vi "delete channel from configuration.vi"(8 "error in":errorcluster, 10 "channel":refnum<class "TBM channel.lvclass">, 11 "Scaling configuration in":refnum<class "Scaling configuration.lvclass">) -> (0 "error out":errorcluster, 3 "Scaling configuration out":refnum<class "Scaling configuration.lvclass">)   [LabVIEW 2013, in "Scaling configuration.lvclass"]
uses:
  Scaling configuration.lvclass
  <vilib>/NI/Tag Bus Module Framework/channel/TBM channel.lvclass
  <vilib>/NI/Tag Bus/tag/tag descriptor.lvclass
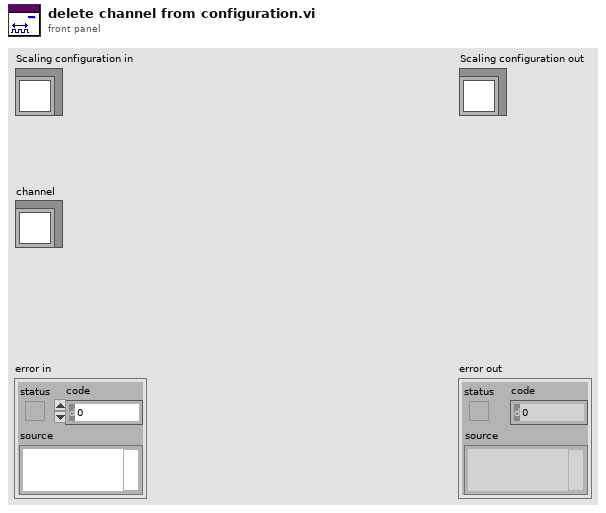
[diagram p1: front panel]
types:
  T1 = typedef "Scaling configuration.lvclass/scale data types.ctl" = enum16{"Double", "Single", "I64", "I32", "I16", "I8", "U64", "U32", "U16", "U8"}
  T2 = cluster{"input channel":refnum<class "TBM channel.lvclass">, "output channel":refnum<class "TBM channel.lvclass">, "input data type":T1, "output data type":T1}[][]
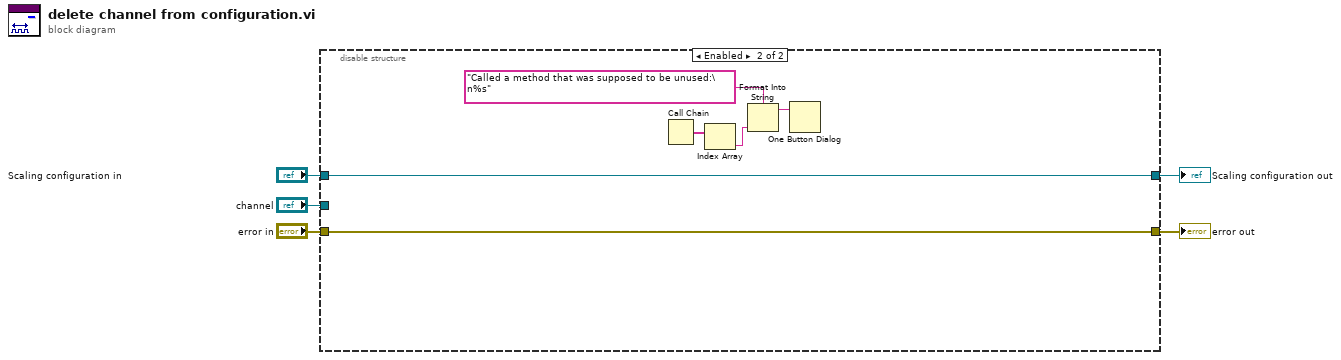
[diagram p0: block diagram]
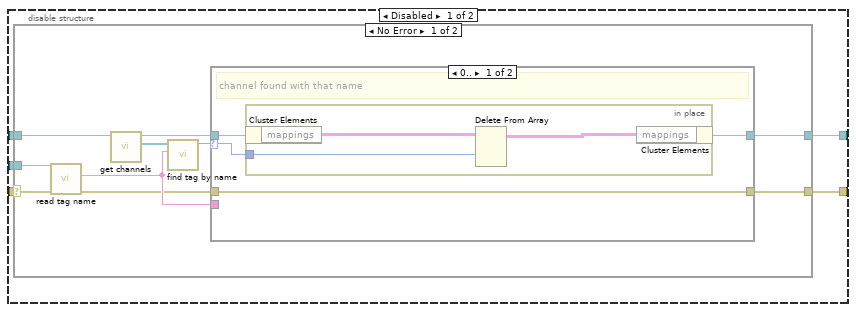
[diagram p2: hidden frame]
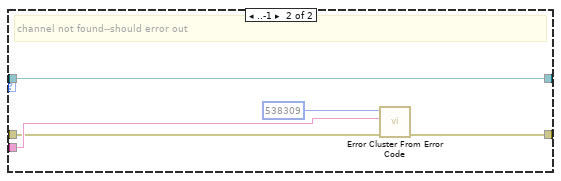
[diagram p3: hidden frame]
diagram:
  n1 = disable-structure shown="Enabled" {
    disable-tunnel: "channel" -> [w10 _]
    disable-tunnel: [w9 w35] -> w4
    disable-tunnel: [w8 w36] -> w3
    disable-tunnel: "Scaling configuration in" -> [w7 w36]
    disable-tunnel: "error in" -> [w6 w35]
    frame Disabled {
      n2 = case shown="No Error" w6 {
        selector: w6 -> [w13 w33]
        tunnel: w10 -> [w19 _]
        tunnel: [w18 w33] -> w9
        tunnel: [w17 w34] -> w8
        tunnel: w7 -> [w16 w34]
        frame No Error {
          n3 = call <vilib>:"read tag name.vi"("error in"=w13, "system tag in"=w19) -> ("error out"=w11:errorcluster, "name"=w12:string)  [unwired: 7 in, 1 out]
          n4 = call-dynamic "get channels.vi"("Scaling configuration in"=w16) -> ("channels"=w15:refnum<class "TBM channel.lvclass">[], "Scaling configuration out"=w20:refnum<class "Scaling configuration.lvclass">)  [unwired: 9 in]
          n5 = call <vilib>:"find tag by name.vi"("name"=w12, "tags in"=w15) -> ("index"=w14:i32)  [unwired: 9 in]
          n6 = case shown="0.." w14 {
            selector: w14 -> [w24 _]
            tunnel: [w21 w32] -> w18
            tunnel: w12 -> [_ w30]
            tunnel: w11 -> [w21 w29]
            tunnel: w20 -> [w23 w28]
            tunnel: [w22 w28] -> w17
            frame 0.. {
              # "channel found with that name"
              n7 = in-place {
                in-place-border: w24 -> [w27]
                n8 = in-place-cluster #1(w23) -> ("mappings"=w26:T2)
                n9 = Delete From Array(array=w26, index (row)=w27) -> (array with subset deleted=w25:T2)  [unwired: 2 in, 1 out]
                n10 = in-place-cluster #1("mappings"=w25) -> (w22:refnum<class "Scaling configuration.lvclass">)
              }
            }
            frame ..-1 {
              # "channel not found--should error out"
              n11 = call <vilib>:"Error Cluster From Error Code.vi"("error in (no error)"=w29, "error message (\"\")"=w30, "error code (0)"=538309) -> ("error out"=w32:errorcluster)  [unwired: 6 in]
            }
          }
        }
        frame Error {
        }
      }
    }
    frame Enabled {
      n12 = Call Chain() -> (call chain=w40:string[])
      n13 = Index Array(array=w40) -> (element=w39:string)  [unwired: 1 in]
      n14 = Format Into String(format string="Called a method that was supposed to be unused:\n%s", w39) -> (resulting string=w37:string)  [unwired: 2 in, 1 out]
      n15 = One Button Dialog(message=w37) -> ()  [unwired: 1 in, 1 out]
    }
  }
  "error out" <- w4
  "Scaling configuration out" <- w3
